vi "PH_gentec_P-Link.PC get and set current Settings for the first Time - 2.vi"(0 "i ref in":refnum<vi>, 2 "VISA resource in":refnum<visa-resource-name>, 3 "Default Head Settings":T1 {"Waveform Averages" items=["None", "2", "4", "8", "16", "32", "64", "128"]; "Trigger Source" items=["Internal", "External"]; "Trigger Polarity" items=["Falling Edge", "Rising Edge"]; "Measurement Mode" items=["other Mode", "Energymode"]}, 5 "error in":errorcluster) -> (14 "i ref out":refnum<vi>, 16 "VISA resource out":refnum<visa-resource-name>, 19 "error out":errorcluster)   [LabVIEW 2014, in "PH_gentec_P-Link.lvlib"]
doc: "This VI gets and sets all current settings for the first time."
uses:
  PH_gentec_P-Link.lvlib
  PH_gentec_M-Link/PH_gentec_M-Link.lvlib
  non_GPL/instr.lib/gentec-M-LINK/Driver/Type Defs/gentec-M-Link.Range Queries.ctl
  PH_gentec_P-Link.Head Settings.ctl
  instr.lib/Gentec-M-Link/Driver/Type Defs/gentec-M-Link.Measurement Mode.ctl
  instr.lib/Gentec-M-Link/gentec-M-Link - Driver.lvlib
  instr.lib/Gentec-M-Link/Driver/Type Defs/gentec-M-Link.Trigger Polarity.ctl
  instr.lib/Gentec-M-Link/Driver/Type Defs/gentec-M-Link.Trigger Source.ctl
  instr.lib/Gentec-M-Link/Driver/Type Defs/gentec-M-Link.Waveform Averages.ctl
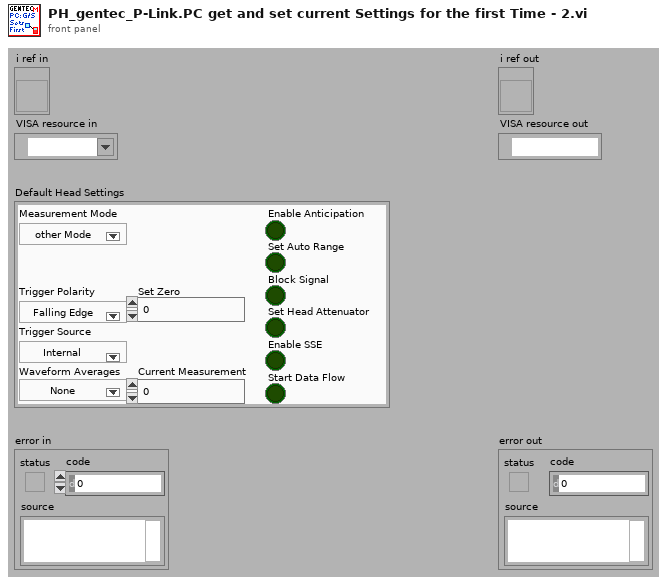
[diagram p1: front panel]
types:
  T1 = typedef "PH_gentec_P-Link.lvlib/PH_gentec_P-Link.Head Settings.ctl" = cluster{"Measurement Mode":T2, "Enable Anticipation":bool, "Set Auto Range":bool, "Block Signal":bool, "Set Head Attenuator":bool, "Enable SSE":bool, "Trigger Polarity":T3, "Trigger Source":T4, "Waveform Averages":T5, "Set Zero":i32, "Current Measurement":i32, "Start Data Flow":bool}
  T2 = typedef "gentec-M-Link - Driver.lvlib/gentec-M-Link.Measurement Mode.ctl" = u16
  T3 = typedef "gentec-M-Link - Driver.lvlib/gentec-M-Link.Trigger Polarity.ctl" = u16
  T4 = typedef "gentec-M-Link - Driver.lvlib/gentec-M-Link.Trigger Source.ctl" = u16
  T5 = typedef "gentec-M-Link - Driver.lvlib/gentec-M-Link.Waveform Averages.ctl" = u16
  T6 = typedef "PH_gentec_P-Link.lvlib/PH_gentec_P-Link.i attribute.ctl" = cluster{"GUI References":cluster{"Wanted Head Settings":refnum<vi>, "Current Head Settings":refnum<vi>, "Set Auto Range":refnum<vi>, "Trigger Polarity":refnum<vi>, "Trigger Source":refnum<vi>, "Waveform Averages":refnum<vi>, "Continuous":refnum<vi>, "get one Value":refnum<vi>}, "Wanted Head Settings":T1, "Current Head Settings":T1}
  T7 = typedef "gentec-M-LINK.lvlib/gentec-M-Link.Range.ctl" = u16
  T8 = typedef "gentec-M-LINK.lvlib/gentec-M-Link.Range Queries.ctl" = string
  T9 = typedef "gentec-M-LINK.lvlib/gentec-M-Link.Waveform Averages.ctl" = u16
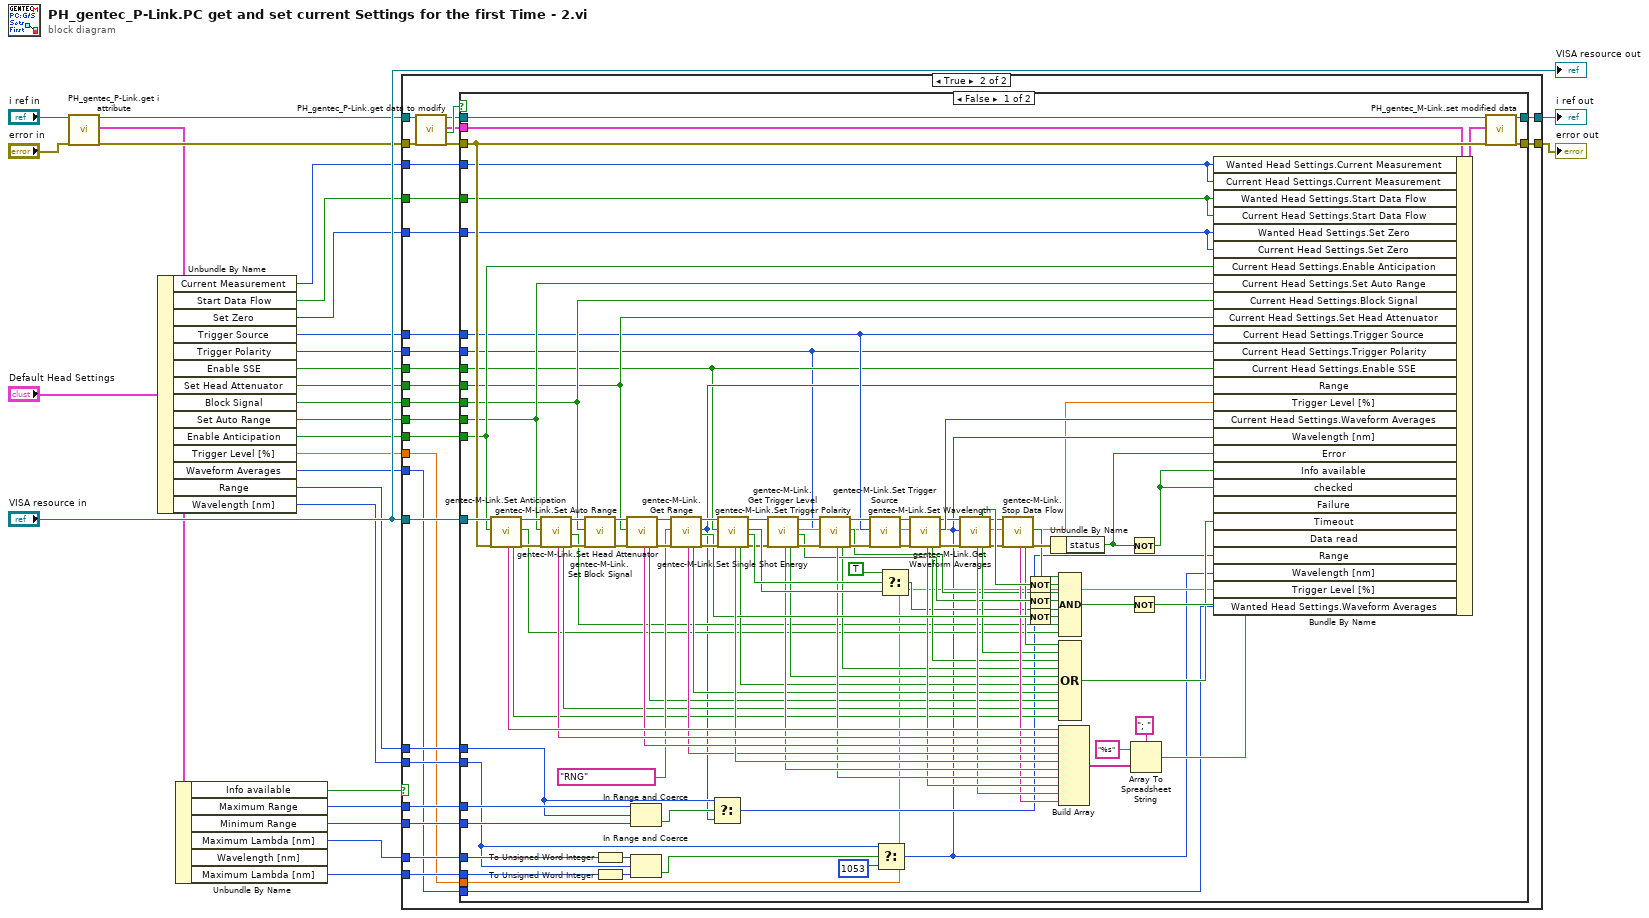
[diagram p0: block diagram]
diagram:
  n1 = call "PH_gentec_P-Link.get i attribute.vi"("i ref in"="i ref in", "error in (no error)"="error in") -> ("i ref out"=w24:refnum<vi>, "i attribute"=w21:T6, "error out"=w22:errorcluster)  [unwired: 15 in]
  n2 = Unbundle By Name("Default Head Settings") -> ("Current Measurement"=w3:i32, "Start Data Flow"=w2:bool, "Set Zero"=w1:i32, "Trigger Source"=w6:T4, "Trigger Polarity"=w7:T3, "Enable SSE"=w10:bool, "Set Head Attenuator"=w11:bool, "Block Signal"=w12:bool, "Set Auto Range"=w13:bool, "Enable Anticipation"=w14:bool, "Trigger Level [%]"=w8:dbl, "Waveform Averages"=w5:T5, "Range"=w9:T7, "Wavelength [nm]"=w4:u16)
  n3 = Unbundle By Name(w21) -> ("Info available"=w20:bool, "Maximum Range"=w19:T7, "Minimum Range"=w18:T7, "Maximum Lambda [nm]"=w17:i32, "Maximum Lambda [nm]"=w16:i32)  [unwired: 1 out]
  n4 = case shown="True" w20 {
    tunnel: [w29 w53] -> w28
    tunnel: [w30 w52] -> w27
    tunnel: "VISA resource in" -> [_ w51]
    tunnel: w24 -> [w30 w50]
    tunnel: w22 -> [w29 w49]
    tunnel: w9 -> [_ w48]
    tunnel: w19 -> [_ w47]
    tunnel: w18 -> [_ w46]
    tunnel: w17 -> [_ w45]
    tunnel: w4 -> [_ w44]
    tunnel: w16 -> [_ w43]
    tunnel: w14 -> [_ w42]
    tunnel: w13 -> [_ w41]
    tunnel: w12 -> [_ w40]
    tunnel: w11 -> [_ w39]
    tunnel: w10 -> [_ w38]
    tunnel: w8 -> [_ w37]
    tunnel: w7 -> [_ w36]
    tunnel: w6 -> [_ w35]
    tunnel: w5 -> [_ w34]
    tunnel: w3 -> [_ w33]
    tunnel: w2 -> [_ w32]
    tunnel: w1 -> [_ w31]
    frame False {
    }
    frame True {
      n5 = call "PH_gentec_P-Link.get data to modify.vi"("i ref in"=w50, "error in (no error)"=w49) -> ("i ref out"=w55:refnum<vi>, "i attribute"=w56:T6, "timed out"=w57:bool, "error out"=w54:errorcluster)  [unwired: 14 in]
      n6 = case shown="False" w57 {
        tunnel: w51 -> [w156 _]
        tunnel: [w159 w161] -> w52
        tunnel: [w158 w160] -> w53
        tunnel: w54 -> [w153 w160]
        tunnel: w55 -> [w157 w161]
        tunnel: w56 -> [w138 _]
        tunnel: w48 -> [w77 _]
        tunnel: w47 -> [w84 _]
        tunnel: w46 -> [w83 _]
        tunnel: w45 -> [w82 _]
        tunnel: w44 -> [w74 _]
        tunnel: w43 -> [w81 _]
        tunnel: w42 -> [w73 _]
        tunnel: w41 -> [w72 _]
        tunnel: w40 -> [w71 _]
        tunnel: w39 -> [w70 _]
        tunnel: w38 -> [w62 _]
        tunnel: w37 -> [w69 _]
        tunnel: w36 -> [w61 _]
        tunnel: w35 -> [w68 _]
        tunnel: w34 -> [w67 _]
        tunnel: w33 -> [w60 _]
        tunnel: w32 -> [w59 _]
        tunnel: w31 -> [w58 _]
        frame False {
          n7 = call "gentec-M-Link.Set Anticipation.vi"("VISA resource In"=w156, "Enable Anticipation"=w73, "error in (no error)"=w153) -> ("Data Read"=w148:string, "Read Timeout"=w95:bool, "VISA resource Out"=w154:refnum<visa-resource-name>, "Success"=w86:bool, "error out"=w152:errorcluster)  [unwired: 12 in]
          n8 = call "gentec-M-Link.Set Auto Range.vi"("VISA resource In"=w154, "Auto Range"=w72, "error in (no error)"=w152) -> ("Data Read"=w147:string, "Read Timeout"=w96:bool, "VISA resource Out"=w155:refnum<visa-resource-name>, "Success"=w87:bool, "error out"=w151:errorcluster)  [unwired: 12 in]
          n9 = call "gentec-M-Link.Set Block Signal.vi"("VISA resource In"=w155, "Block Signal"=w71, "error in (no error)"=w151) -> ("VISA resource Out"=w150:refnum<visa-resource-name>, "error out"=w149:errorcluster)  [unwired: 15 in]
          n10 = To Unsigned Word Integer(number=w82) -> (unsigned 16bit integer=w80:u16)
          n11 = To Unsigned Word Integer(number=w81) -> (unsigned 16bit integer=w79:u16)
          n12 = call "gentec-M-Link.Set Head Attenuator.vi"("VISA resource In"=w150, "Set Head Attenuator"=w70, "error in (no error)"=w149) -> ("Data Read"=w146:string, "Read Timeout"=w97:bool, "VISA resource Out"=w133:refnum<visa-resource-name>, "error out"=w131:errorcluster)  [unwired: 11 in, 2 out]
          n13 = In Range and Coerce(upper limit=w84, x=w77, lower limit=w83) -> (In Range?=w78:bool)  [unwired: 1 out]
          n14 = In Range and Coerce(upper limit=w80, x=w74, lower limit=w79) -> (In Range?=w75:bool)  [unwired: 1 out]
          n15 = call "gentec-M-Link.Get Range.vi"("VISA resource In"=w133, "Range Queries"=T8 "RNG", "error in (no error)"=w131) -> ("Data Read"=w128:string, "Read Timeout"=w98:bool, "VISA resource Out"=w132:refnum<visa-resource-name>, "Range"=w63:T7, "Error"=w127:bool, "error out"=w130:errorcluster)  [unwired: 11 in]
          n16 = Select(t=w77, s=w78, f=w63) -> (s? t:f=w76:T7)
          n17 = call "gentec-M-Link.Set Single Shot Energy.vi"("VISA resource In"=w132, "Enable Single Shot Energy"=w62, "error in (no error)"=w130) -> ("Data Read"=w145:string, "Read Timeout"=w99:bool, "VISA resource Out"=w126:refnum<visa-resource-name>, "Success"=w140:bool, "no Thermopyle Head"=w141:bool, "error out"=w125:errorcluster)  [unwired: 11 in]
          n18 = call "gentec-M-Link.Get Trigger Level.vi"("VISA resource In"=w126, "error in (no error)"=w125) -> ("Data Read"=w124:string, "Read Timeout"=w100:bool, "VISA resource Out"=w121:refnum<visa-resource-name>, "Trigger Level [%]"=w64:dbl, "Error"=w110:bool, "error out"=w123:errorcluster)  [unwired: 12 in]
          n19 = call "gentec-M-Link.Set Trigger Polarity.vi"("VISA resource In"=w121, "Trigger Polarity"=w61, "error in (no error)"=w123) -> ("Data Read"=w119:string, "Read Timeout"=w101:bool, "VISA resource Out"=w120:refnum<visa-resource-name>, "Success"=w91:bool, "error out"=w122:errorcluster)  [unwired: 12 in]
          n20 = call "gentec-M-Link.Set Trigger Source.vi"("VISA resource In"=w120, "Trigger Source"=w68, "error in (no error)"=w122) -> ("VISA resource Out"=w118:refnum<visa-resource-name>, "error out"=w117:errorcluster)  [unwired: 15 in]
          n21 = Select(t=w74, s=w75, f=u16 1053) -> (s? t:f=w65:u16)
          n22 = Select(t=TRUE, s=w141, f=w140) -> (s? t:f=w89:bool)
          n23 = call "gentec-M-Link.Get Waveform Averages.vi"("VISA resource In"=w118, "error in (no error)"=w117) -> ("Data Read"=w116:string, "Read Timeout"=w102:bool, "VISA resource Out"=w113:refnum<visa-resource-name>, "Waveform Averages"=w115:T9, "error out"=w114:errorcluster)  [unwired: 13 in]
          n24 = call "gentec-M-Link.Set Wavelength.vi"("VISA resource In"=w113, "Lambda"=w65, "error in (no error)"=w114) -> ("Data Read"=w112:string, "Error"=w111:bool, "Read Timeout"=w103:bool, "VISA resource Out"=w107:refnum<visa-resource-name>, "error out"=w109:errorcluster)  [unwired: 8 in, 4 out]
          n25 = call "gentec-M-Link.Stop Data Flow.vi"("VISA resource In"=w107, "error in (no error)"=w109) -> ("Data Read"=w105:string, "Read Timeout"=w104:bool, "Success"=w93:bool, "error out"=w108:errorcluster)  [unwired: 13 in, 1 out]
          n26 = Not(x=w111) -> (.not. x?=w92:bool)
          n27 = Not(x=w110) -> (.not. x?=w90:bool)
          n28 = Not(x=w127) -> (.not. x?=w88:bool)
          n29 = Unbundle By Name(w108) -> ("status"=w135:bool)
          n30 = Compound Arithmetic op=AND(w93, w92, w91, w90, w89, w88, w87, w86) -> (w85:bool)
          n31 = Compound Arithmetic op=OR(w104, w103, w102, w101, w100, w99, w98, w97, w96, w95) -> (w94:bool)
          n32 = Build Array(w148, w147, w146, w128, w145, w124, w119, w116, w112, w105) -> (w142:string[])
          n33 = Not(x=w135) -> (.not. x?=w106:bool)
          n34 = Not(x=w85) -> (.not. x?=w136:bool)
          n35 = Array To Spreadsheet String(delimiter (Tab)="; ", array=w142, 3:"%s" ("format string")) -> (spreadsheet string=w137:string)
          n36 = Bundle By Name(cluster=w138, "Wanted Head Settings.Current Measurement"=w60, "Current Head Settings.Current Measurement"=w60, "Wanted Head Settings.Start Data Flow"=w59, "Current Head Settings.Start Data Flow"=w59, "Wanted Head Settings.Set Zero"=w58, "Current Head Settings.Set Zero"=w58, "Current Head Settings.Enable Anticipation"=w73, "Current Head Settings.Set Auto Range"=w72, "Current Head Settings.Block Signal"=w71, "Current Head Settings.Set Head Attenuator"=w70, "Current Head Settings.Trigger Source"=w68, "Current Head Settings.Trigger Polarity"=w61, "Current Head Settings.Enable SSE"=w62, "Range"=w63, "Trigger Level [%]"=w64, "Current Head Settings.Waveform Averages"=w115, "Wavelength [nm]"=w65, "Error"=w135, "Info available"=w106, "checked"=w106, "Failure"=w136, "Timeout"=w94, "Data read"=w137, "Range"=w76, "Wavelength [nm]"=w65, "Trigger Level [%]"=w69, "Wanted Head Settings.Waveform Averages"=w67) -> (w134:T6)
          n37 = call "PH_gentec_M-Link.set modified data.vi"("i ref in"=w157, "i attribute"=w134, "error in (no error)"=w153) -> ("i ref out"=w159:refnum<vi>, "error out"=w158:errorcluster)  [unwired: 15 in]
        }
        frame True {
        }
      }
    }
  }
  "error out" <- w28
  "i ref out" <- w27
  "VISA resource out" <- "VISA resource in"
